vi "Encoder Test.vi"() -> ()   [LabVIEW 2021]
panel:
  out "Mes Pos (mm)":cluster{dbl, dbl}(graph)
  out "RPM":cluster{dbl, dbl}(graph)
  in  "stop":bool
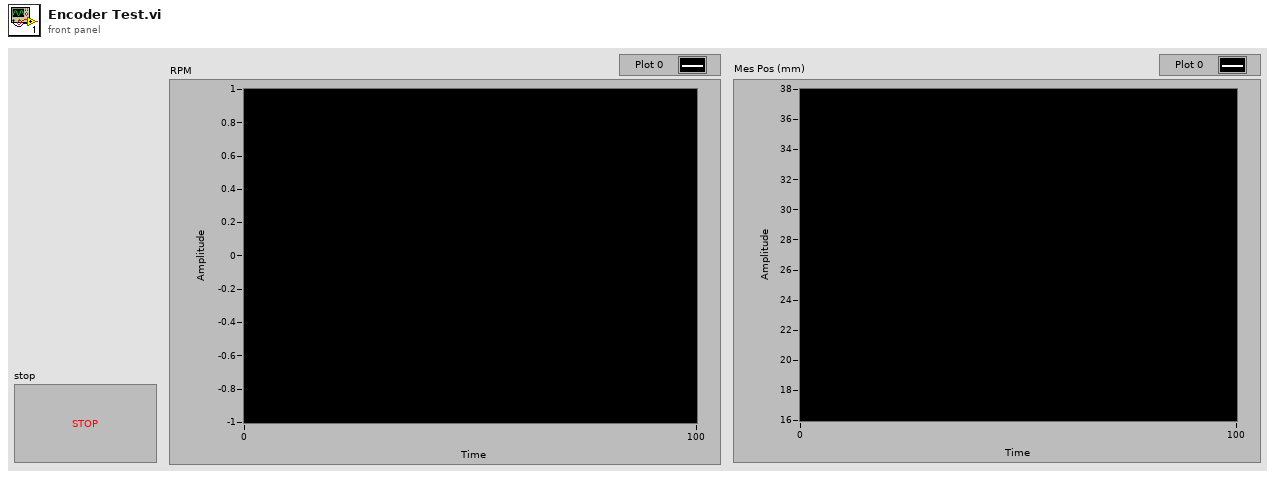
[diagram p1: front panel]
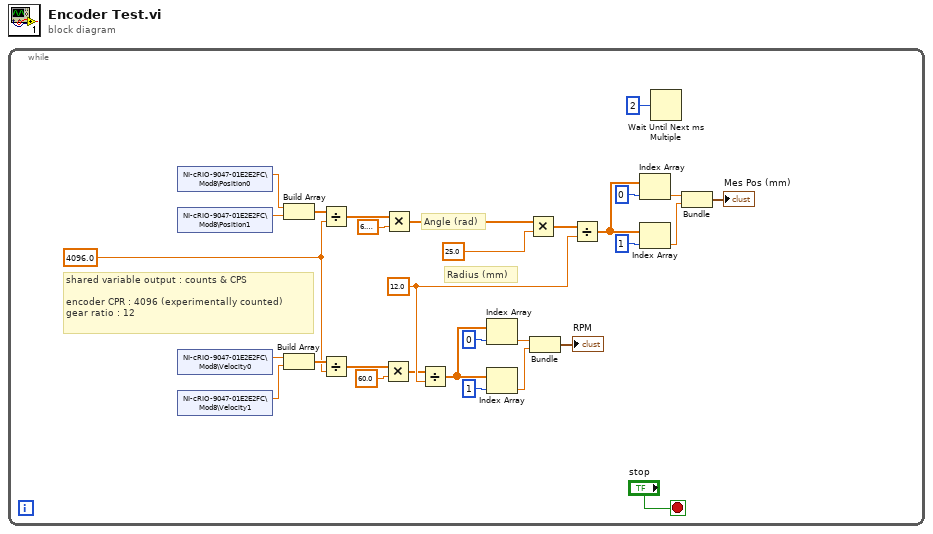
[diagram p0: block diagram]
diagram:
  n1 = while {
    stop <- "stop" stop-if-true
    w14 = 12.0 ("y")
    w18 = 4096.0 ("y")
    # "Radius (mm)"
    # "Angle (rad)"
    # "shared variable output : counts & CPS\n\nencoder CPR : 4096 (experimentally counted)\ngear ratio : 12"
    n2 = shared-variable "NI-cRIO-9047-01E2E2FC\\Mod8\\Position0"() -> (w22:dbl)  [unwired: 1 in, 1 out]
    n3 = shared-variable "NI-cRIO-9047-01E2E2FC\\Mod8\\Position1"() -> (w21:dbl)  [unwired: 1 in, 1 out]
    n4 = shared-variable "NI-cRIO-9047-01E2E2FC\\Mod8\\Velocity0"() -> (w26:dbl)  [unwired: 1 in, 1 out]
    n5 = shared-variable "NI-cRIO-9047-01E2E2FC\\Mod8\\Velocity1"() -> (w25:dbl)  [unwired: 1 in, 1 out]
    n6 = Build Array(w22, w21) -> (w23:dbl[])
    n7 = Build Array(w26, w25) -> (w24:dbl[])
    n8 = Divide(x=w23, y=w18) -> (x/y=w20:dbl[])
    n9 = Divide(x=w24, y=w18) -> (x/y=w28:dbl[])
    n10 = Multiply(x=w28, y=60.0) -> (x*y=w13:dbl[])
    n11 = Multiply(x=w20, y=6.283185307179586) -> (x*y=w17:dbl[])
    n12 = Divide(x=w13, y=w14) -> (x/y=w4:dbl[])
    n13 = Index Array(array=w4, index=0) -> (element=w3:dbl)
    n14 = Index Array(array=w4, index=1) -> (element=w2:dbl)
    n15 = Multiply(x=w17, y=25.0) -> (x*y=w15:dbl[])
    n16 = Bundle(w3, w2) -> (→"RPM":cluster{dbl, dbl})  [unwired: 1 in]
    n17 = Divide(x=w15, y=w14) -> (x/y=w8:dbl[])
    n18 = Index Array(array=w8, index=0) -> (element=w7:dbl)
    n19 = Index Array(array=w8, index=1) -> (element=w6:dbl)
    n20 = Wait Until Next ms Multiple(millisecond multiple=u32 2) -> ()  [unwired: 1 out]
    n21 = Bundle(w7, w6) -> (→"Mes Pos (mm)":cluster{dbl, dbl})  [unwired: 1 in]
  }
